vi "GetHelp.vi"(0 "XRef":T32, 1 "Point":T31, 2 "State In":T13={"BlockNodeState"={"Terminal Data"=[], "Instance Name"="", "Type Name"="", "Draw Style"=0, "Connector Pane Pattern"=0, "Flags"=0, "Grown Terminal List Order"=[], "Image"={"image type"=0, "image depth"=0, "image"=[], "mask"=[], "colors"=[], "Rectangle"={"left"=0, "top"=0, "right"=0, "bottom"=0}}}, "stateInfo"={"Data storage parameters"={"Name"="", "Format"="TDM", "Connection string"="", "use default"=TRUE}, "Object type"="root", "Selected properties"=[], "Object definitions"=[], "Refnum input wired"=enum."<none>", "Parent object type"="", "Parent object child property"="", "Channel options"=enum."Replace values at index", "PendingCommand"=enum."<none>", "Node style"=enum."Classic", "Only child objects"=FALSE, "TermSpecs"=[], "objectTypeWired"="", "Dynamic format"=FALSE, "Overwrite options"=enum."open or create", "Parameters"=variant, "Format"="", "Node type"=enum."UPDATE", "ImplicitExplicit"=enum."explicit", "Channel type"=enum."Waveform", "Use object with same name"=FALSE, "Show channel terminal"=FALSE, "LabVIEW Version"="", "DataTerminals"=enum."Express", "Size to text"=FALSE, "selected nodes in"=[]}} {"BlockNodeState"."Draw Style" items=["FunctionBlock", "ExpressVI", "Variable", "Elemental I/O", "32x32 Icon", "FunctionBlockCompact"]; "BlockNodeState"."Terminal Data"."Terminal Flags" format="%.0b"}) -> (14 "Standard Help Info":T11, 15 "Detailed Help Info":T8, 16 "Subitem Help Info":T2, 17 "Use Detailed Help?":T1, 18 "Use Subitem Help?":T1)   [LabVIEW 2020, in "Get Properties.xnode"]
doc: "Reads property values from a file, channel group, or channel. If you configure this Express VI before you wire a refnum to <B>storage refnum</B>, the configuration might change depending on the refnum you wire. For example, if you configure this Express VI for a channel and then wire a channel group refnum, this Express VI returns broken wires on the block diagram because the same properties are not available for a channel group."
uses:
  <vilib>/Platform/storage/lvStorage.llb/xStorage/Get Properties/Get Properties.xnode
  <vilib>/XNodeSupport/XNodeXNodeRef.ctl
  <vilib>/XNodeSupport/XNodePoint.ctl
  <vilib>/XNodeSupport/XNodeInt.ctl
  <vilib>/Platform/storage/lvStorage.llb/xStorage/Get Properties/State.ctl
  <vilib>/BlockNodeSupport/BlockNodeState.ctl
  <vilib>/BlockNodeSupport/TerminalData.ctl
  <vilib>/picture/picture.llb/imagedata.ctl
  <vilib>/Platform/storage/lvStorage.llb/dataStorageParams.ctl
  <vilib>/Platform/storage/lvStorage.llb/_selectedProp.ctl
  <vilib>/Platform/storage/lvStorage.llb/dataModel.ctl
  <vilib>/Platform/storage/Storage.llb/usiTypeDef.ctl
  <vilib>/Platform/storage/Storage.llb/usiPropDef.ctl
  <vilib>/express/express shared/ex_EditUserDefinedProperties/usiDataType.ctl
  <vilib>/Platform/storage/Storage.llb/specialProperties.ctl
  <vilib>/Platform/storage/Storage.llb/usiOverwriteOptions.ctl
  <vilib>/Platform/storage/lvStorage.llb/TerminalDef.ctl
  <vilib>/Platform/storage/lvStorage.llb/_TerminalStyle.ctl
  <vilib>/Utility/XNodeSupport.llb/XRect32.ctl
  <vilib>/Platform/storage/Storage.llb/usiSequenceRepresentation.ctl
  <vilib>/Platform/storage/lvStorage.llb/channelType.ctl
  <vilib>/Platform/storage/lvStorage.llb/_dataTerminals.ctl
  <vilib>/XNodeSupport/XNodeStandardHelpInfo.ctl
  <vilib>/XNodeSupport/XNodeString.ctl
  <vilib>/XNodeSupport/XNodePath.ctl
  <vilib>/XNodeSupport/XNodeDetailedHelpInfo.ctl
  <vilib>/XNodeSupport/XNodeImage.ctl
  <vilib>/XNodeSupport/XNodeRect32.ctl
  <vilib>/XNodeSupport/XNodeTerms.ctl
  <vilib>/XNodeSupport/XNodeTerm.ctl
  <vilib>/XNodeSupport/XNodeVariant.ctl
  <vilib>/XNodeSupport/XNodeBool.ctl
  <vilib>/XNodeSupport/XNodeSubitemHelpInfo.ctl
  <vilib>/XNodeSupport/NI_XNodeSupport.lvlib
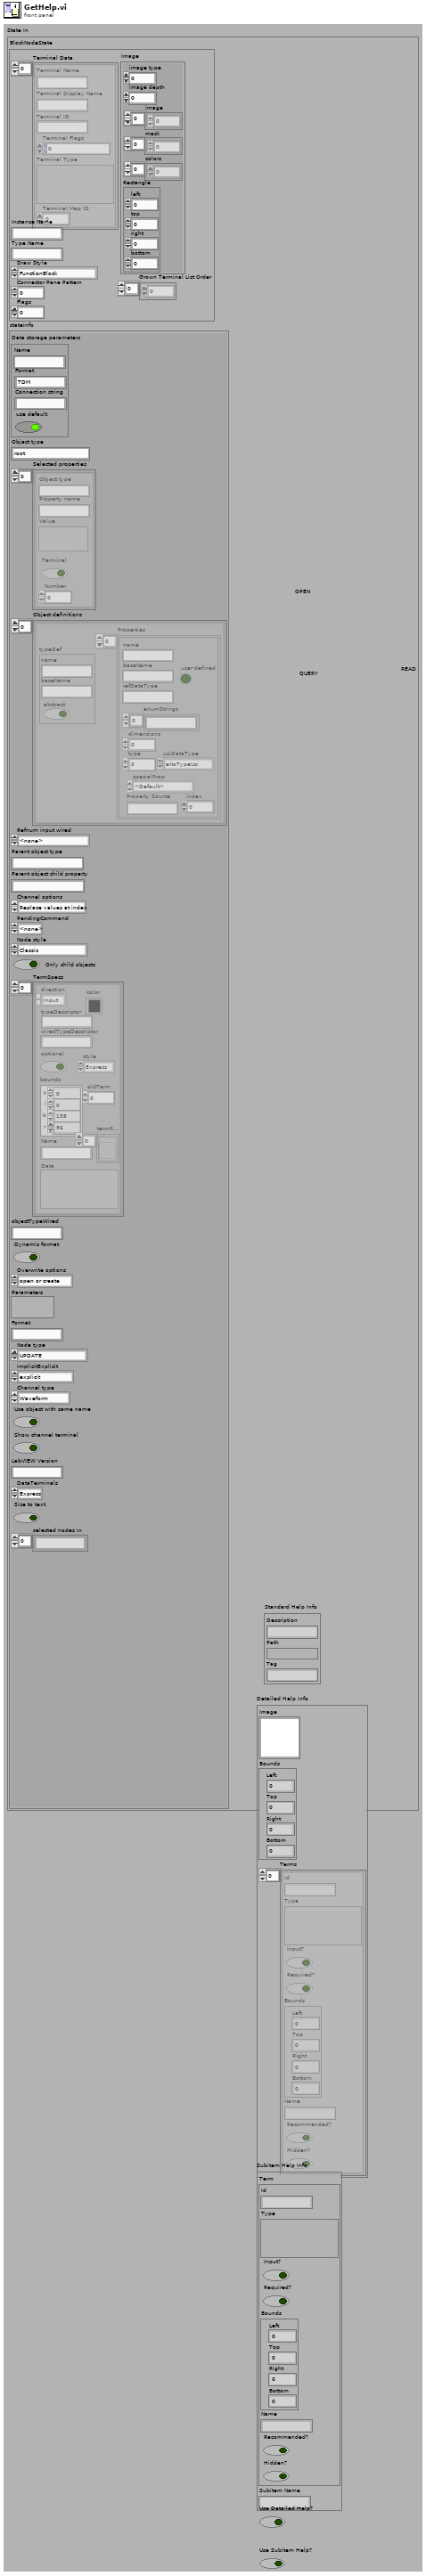
[diagram p1: front panel]
types:
  T1 = typedef "NI_XNodeSupport.lvlib/XNodeBool.ctl" = bool
  T2 = typedef "NI_XNodeSupport.lvlib/XNodeSubitemHelpInfo.ctl" = cluster{"Term":T3, "Subitem Name":T4}
  T3 = typedef "NI_XNodeSupport.lvlib/XNodeTerm.ctl" = cluster{"Id":T4, "Type":T5, "Input?":T1, "Required?":T1, "Bounds":T6, "Name":T4, "Recommended?":T1, "Hidden?":T1}
  T4 = typedef "NI_XNodeSupport.lvlib/XNodeString.ctl" = string
  T5 = typedef "NI_XNodeSupport.lvlib/XNodeVariant.ctl" = variant
  T6 = typedef "NI_XNodeSupport.lvlib/XNodeRect32.ctl" = cluster{"Left":T7, "Top":T7, "Right":T7, "Bottom":T7}
  T7 = typedef "NI_XNodeSupport.lvlib/XNodeInt.ctl" = i32
  T8 = typedef "NI_XNodeSupport.lvlib/XNodeDetailedHelpInfo.ctl" = cluster{"Image":T9, "Bounds":T6, "Terms":T10}
  T9 = typedef "NI_XNodeSupport.lvlib/XNodeImage.ctl" = picture
  T10 = typedef "NI_XNodeSupport.lvlib/XNodeTerms.ctl" = T3[]
  T11 = typedef "NI_XNodeSupport.lvlib/XNodeStandardHelpInfo.ctl" = cluster{"Description":T4, "Path":T12, "Tag":T4}
  T12 = typedef "NI_XNodeSupport.lvlib/XNodePath.ctl" = path
  T13 = typedef "Get Properties.xnode/State.ctl" = cluster{"BlockNodeState":T14, "stateInfo":cluster{"Data storage parameters":T17, "Object type":string, "Selected properties":T18[], "Object definitions":T19[], "Refnum input wired":enum16{"Storage", "Generic object", "Typed object", "<none>"}, "Parent object type":string, "Parent object child property":string, "Channel options":T24, "PendingCommand":enum16{"<none>", "SelPopUp", "Init"}, "Node style":enum16{"Classic", "Express"}, "Only child objects":bool, "TermSpecs":T25[], "objectTypeWired":string, "Dynamic format":bool, "Overwrite options":enum16{"open", "open or create", "create or replace", "create", "open (read only)"}, "Parameters":variant, "Format":string, "Node type":enum16{"UPDATE", "READ", "QUERY", "CREATE CHILD", "CREATE", "CONNECT", "DISCONNECT"}, "ImplicitExplicit":T28, "Channel type":T29, "Use object with same name":bool, "Show channel terminal":bool, "LabVIEW Version":string, "DataTerminals":T30, "Size to text":bool, "selected nodes in":string[]}}
  T14 = typedef "BlockNodeState.ctl" = cluster{"Terminal Data":T15[], "Instance Name":string, "Type Name":string, "Draw Style":i32, "Connector Pane Pattern":i32, "Flags":i32, "Grown Terminal List Order":i32[], "Image":T16}
  T15 = typedef "TerminalData.ctl" = cluster{"Terminal Name":string, "Terminal Display Name":string, "Terminal ID":string, "Terminal Flags":i32, "Terminal Type":variant, "Terminal Map ID":i32}
  T16 = typedef "imagedata.ctl" = cluster{"image type":i32, "image depth":i32, "image":u8[], "mask":u8[], "colors":u32[], "Rectangle":cluster{"left":i16, "top":i16, "right":i16, "bottom":i16}}
  T17 = typedef "dataStorageParams.ctl" = cluster{"Name":string, "Format":string, "Connection string":string, "use default":bool}
  T18 = typedef "_selectedProp.ctl" = cluster{"Object type":string, "Property name":string, "Value":variant, "Terminal":bool, "Number":i32}
  T19 = typedef "dataModel.ctl" = cluster{"typeDef":T20, "Properties":T21[]}
  T20 = typedef "usiTypeDef.ctl" = cluster{"name":string, "baseName":string, "abstract":bool}
  T21 = typedef "usiPropDef.ctl" = cluster{"name":string, "baseName":string, "refDataType":string, "dimensions":i32, "type":i32, "user defined":bool, "enumStrings":string[], "usiDataType":T22, "specialProp":T23, "Property Source":string, "index":i32}
  T22 = typedef "usiDataType.ctl" = enum16{"eNoTypeUsi", "eInt8Usi", "eInt16Usi", "eInt32Usi", "eInt64Usi", "eUInt8Usi", "eUInt16Usi", "eUInt32Usi", "eUInt64Usi", "eFloat32Usi", "eFloat64Usi", "- 0", "- 1", "- 2", "- 3", "- 4", "- 5", "- 6", "- 7", "- 8", "- 9", "eString8Usi", "eString16Usi", "eStringUsi", "eEnumUsi", "- 10", "- 11", "- 12", "- 13", "- 14", "eTimeUsi", "- 15", "- 16", "- 17", "- 18", "- 19", "- 20", "- 21", "- 22", "- 23", "eInstanceUsi", "eStoreUsi"}
  T23 = typedef "specialProperties.ctl" = enum16{"<Default>", "Channel Values", "AppendReplace", "ChannelFlags", "ValueFlags", "ImplicitExplicit", "InsertIndex", "ValuesCount", "ComparisonOperator", "Cluster", "DAQmx Channel"}
  T24 = typedef "usiOverwriteOptions.ctl" = enum16{"Append values", "Replace values at index", "Replace all values", "Append if timeline aligns"}
  T25 = typedef "TerminalDef.ctl" = cluster{"direction":enum16{"Input", "Output"}, "typeDescriptor":string, "color":u32, "oldTerm":i32, "style":T26, "optional":bool, "bounds":T27, "termRefs":refnum<vi>[], "Name":string, "Data":variant, "wiredTypeDescriptor":string}
  T26 = typedef "_TerminalStyle.ctl" = enum16{"Express", "Collapsed", "Internal"}
  T27 = typedef "XRect32.ctl" = cluster{"t":i32, "l":i32, "b":i32, "r":i32}
  T28 = typedef "usiSequenceRepresentation.ctl" = enum16{"explicit", "implicit"}
  T29 = typedef "channelType.ctl" = enum16{"Waveform", "Array of Double", "Array of String", "DDT", "Array of UInt8", "Array of Int16", "Array of Int32", "Array of Single", "Array of DateTime", "Array of Waveform", "none", "DateTime", "String", "Double", "Single", "UInt8", "Int16", "Int32"}
  T30 = typedef "_dataTerminals.ctl" = enum16{"Express", "Cluster"}
  T31 = typedef "NI_XNodeSupport.lvlib/XNodePoint.ctl" = cluster{"H":T7, "V":T7}
  T32 = typedef "NI_XNodeSupport.lvlib/XNodeXNodeRef.ctl" = refnum<vi>
  T33 = cluster{"Description":string, "Help.Path":path, "Help.Tag":string}
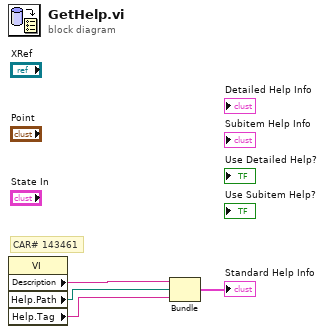
[diagram p0: block diagram]
diagram:
  # "CAR# 143461"
  n1 = property class="VI"() -> ("Description"=w3:string, "Help.Path"=w2:path, "Help.Tag"=w1:string)  [unwired: 2 in, 2 out]
  n2 = Bundle("Description"=w3, "Help.Path"=w2, "Help.Tag"=w1) -> (→"Standard Help Info":T33)  [unwired: 1 out]
